vi "FindConstants.vi"() -> ()   [LabVIEW 2022 SP3]
panel:
  out "In focal Zone?":bool
  out "r":dbl format="%.2f"
  out "rn values":dbl[](array[numeric]) format="%.2f"
  in  "strip":cluster{"radius":dbl, "h":dbl, "w":dbl}={"radius"=10.0, "h"=5.0, "w"=4.0} {"radius" format="%.2f"; "w" format="%.2f"; "h" format="%.2f"}
  in  "P":cluster{"x":dbl, "y":dbl, "z":dbl}={"x"=-4.0, "y"=0.0, "z"=4.0} {"x" format="%.2f"; "z" format="%.2f"; "y" format="%.2f"}
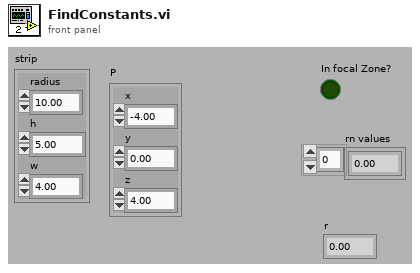
[diagram p1: front panel]
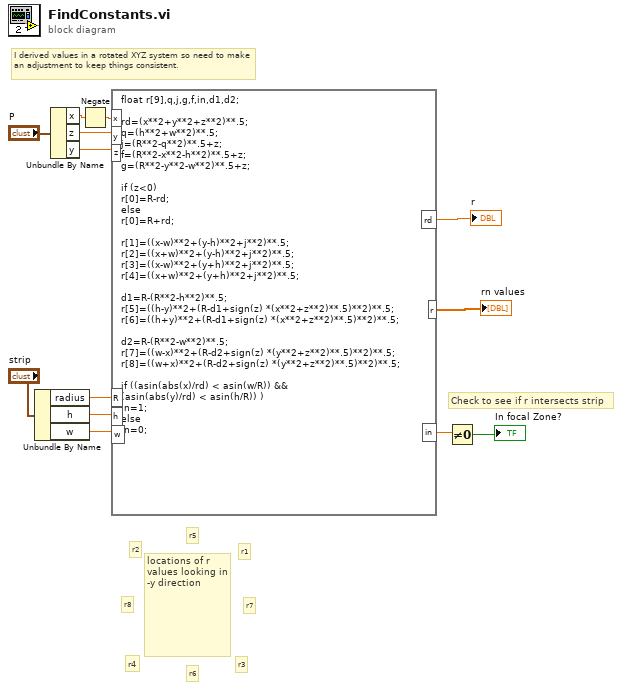
[diagram p0: block diagram]
diagram:
  # "r8"
  # "r7"
  # "r6"
  # "r5"
  # "r4"
  # "r3"
  # "r2"
  # "r1"
  # "locations of r values looking in -y direction"
  # "Check to see if r intersects strip"
  # "I derived values in a rotated XYZ system so need to make an adjustment to keep things consistent."
  n1 = Unbundle By Name("strip") -> ("radius"=w8:dbl, "h"=w7:dbl, "w"=w6:dbl)
  n2 = Unbundle By Name("P") -> ("x"=w12:dbl, "z"=w11:dbl, "y"=w10:dbl)
  n3 = Negate(x=w12) -> (-x=w3:dbl)
  n4 = formula code="float r[9],q,j,g,f,in,d1,d2;\n\nrd=(x**2+y**2+z**2)**.5;\nq=(h**2+w**2)**.5;\nj=(R**2-q**2)**.5+z;\nf=(R**2-x**2-h**2)**.5+z;\ng=(R**2-y**2-w**2)**.5+z;\n\nif (z<0) \nr[0]=R-rd;\nelse\nr[0]=R+rd;\n\nr[1]=((x-w)**2+(y-h)**2+j**2)**.5;\nr[2]=((x+w)**2+(y-h)**2+j**2)**.5;\nr[3]=((x-w)**2+(y+h)**2+j**2)**.5;\nr[4]=((x+w)**2+(y+h)**2+j**2)**.5;\n\nd1=R-(R**2-h**2)**.5;\nr[5]=((h-y)**2+(R-d1+sign(z)\t*(x**2+z**2)**.5)**2)**.5;\nr[6]=((h+y)**2+(R-d1+sign(z)\t*(x**2+z**2)**.5)**2)**.5;\n\nd2=R-(R**2-w**2)**.5;\nr[7]=((w-x)**2+(R-d2+sign(z)\t*(y**2+z**2)**.5)**2)**.5;\nr[8]=((w+x)**2+(R-d2+sign(z)\t*(y**2+z**2)**.5)**2)**.5;\n\nif ((asin(abs(x)/rd) < asin(w/R)) &&\n(asin(abs(y)/rd) < asin(h/R)) )\nin=1;\nelse\nin=0;"("z"=w10, "x"=w3, "y"=w11, "R"=w8, "w"=w6, "h"=w7) -> ("in"=w1:dbl, "r"=→"rn values":dbl[], "rd"=→"r":dbl)
  n5 = Not Equal To 0?(x=w1) -> (x != 0?=→"In focal Zone?":bool)
